vi "LoadZstackImages.vi"(0 "Experiment folder path OR Z-stack folder path":path, 11 "Error In":errorcluster) -> (1 "Number of Files":i32, 2 "All outputs":T2, 3 "AOL Z Planes":dbl[](array[numeric]), 4 "Red Image Array":T1[](array[typedef]), 6 "Green Image Array":T1[](array[typedef]), 8 "Motor Z planes":dbl[](array[numeric]), 10 "AOL Z Planes (norm)":dbl[](array[numeric]), 12 "RedMaxZ":T1, 14 "GreenMaxZ":T1, 15 "Error Out":errorcluster)   [LabVIEW 2020]
uses:
  <vilib>/vision/Image Controls.llb/IMAQ Image.ctl
  <vilib>/vision/NI_Vision_Development_Module.lvlib
panel:
  out "error IO":errorcluster
  out "Green":path[](array[path])
  out "Red":path[](array[path])
  out "GreenMaxZ":T1
  out "RedMaxZ":T1
  out "GreenImageArray":T1[](array[typedef])
  out "RedImageArray":T1[](array[typedef])
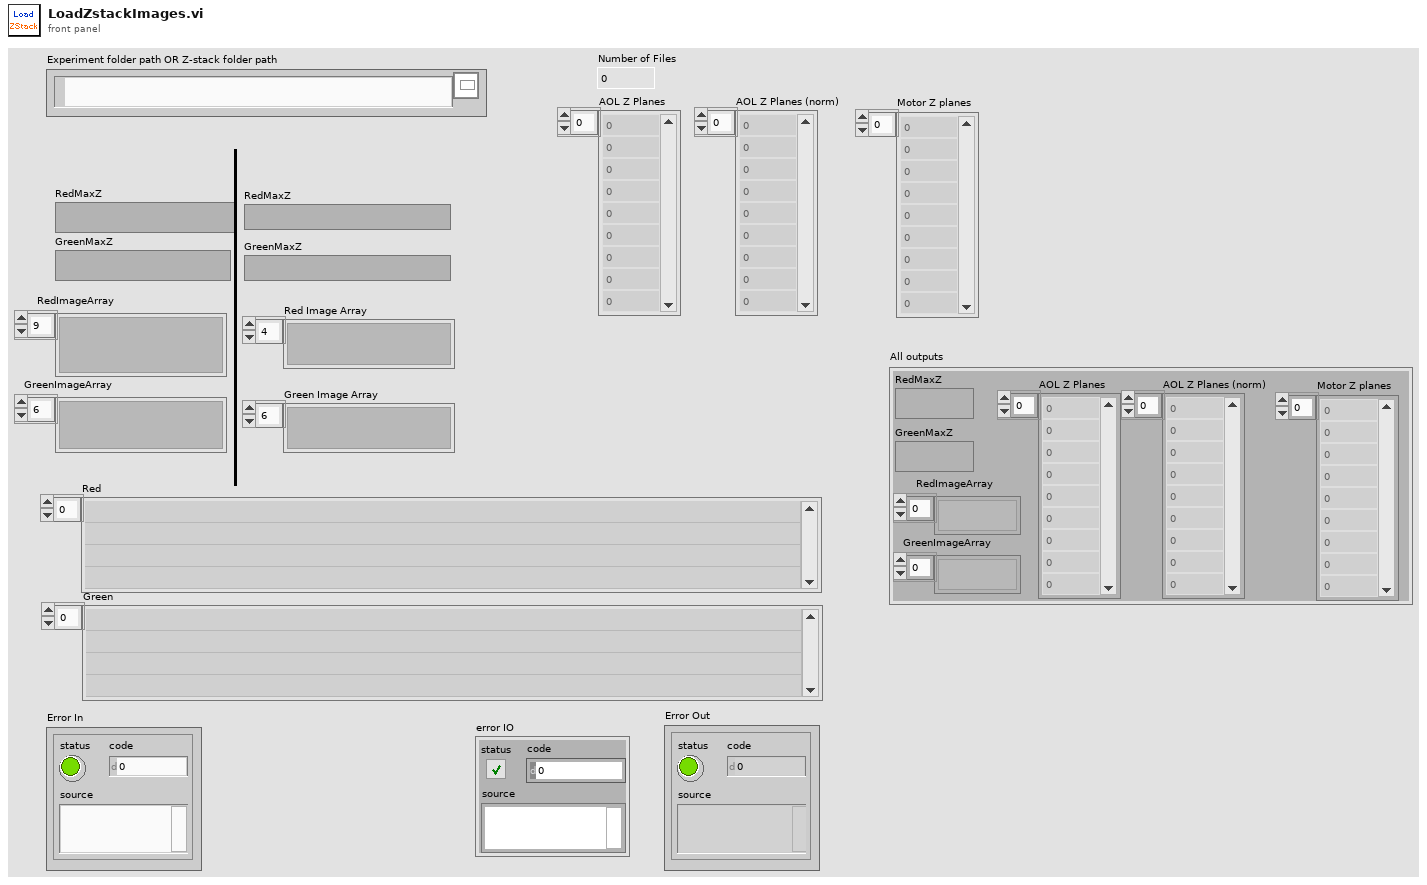
[diagram p1: front panel]
types:
  T1 = typedef "IMAQ Image.ctl" = refnum<image>
  T2 = cluster{"RedImageArray":T1[], "GreenImageArray":T1[], "RedMaxZ":T1, "GreenMaxZ":T1, "AOL Z Planes":dbl[], "AOL Z Planes (norm)":dbl[], "Motor Z planes":dbl[]}
  T3 = typedef "Fixed strings.ctl" = cluster{"ROI file name":string, "Normalised ROI file name":string, "Zplane Pockels values file name":string, "Functional data folder name":string, "Experiment Header file name":string, "Z-stack images folder name":string, "Groups setup rel. path":string, "Groups text file rel. path":string, "TDMS files folder name (F.img)":string, "TDMS files folder name (V.acq)":string, "TDMS files folder name (Pl.acq)":string, "Cycle rel times sequence file":string, "Dynamically called VIs folder name":string, "Time Series folder base name":string}
  T4 = enum32{"Average", "Min", "Max", "Clear  if < ", "Clear  if < or =", "Clear  if =", "Clear  if > or =", "Clear  if >"}
  T5 = typedef "Image Type" = u32
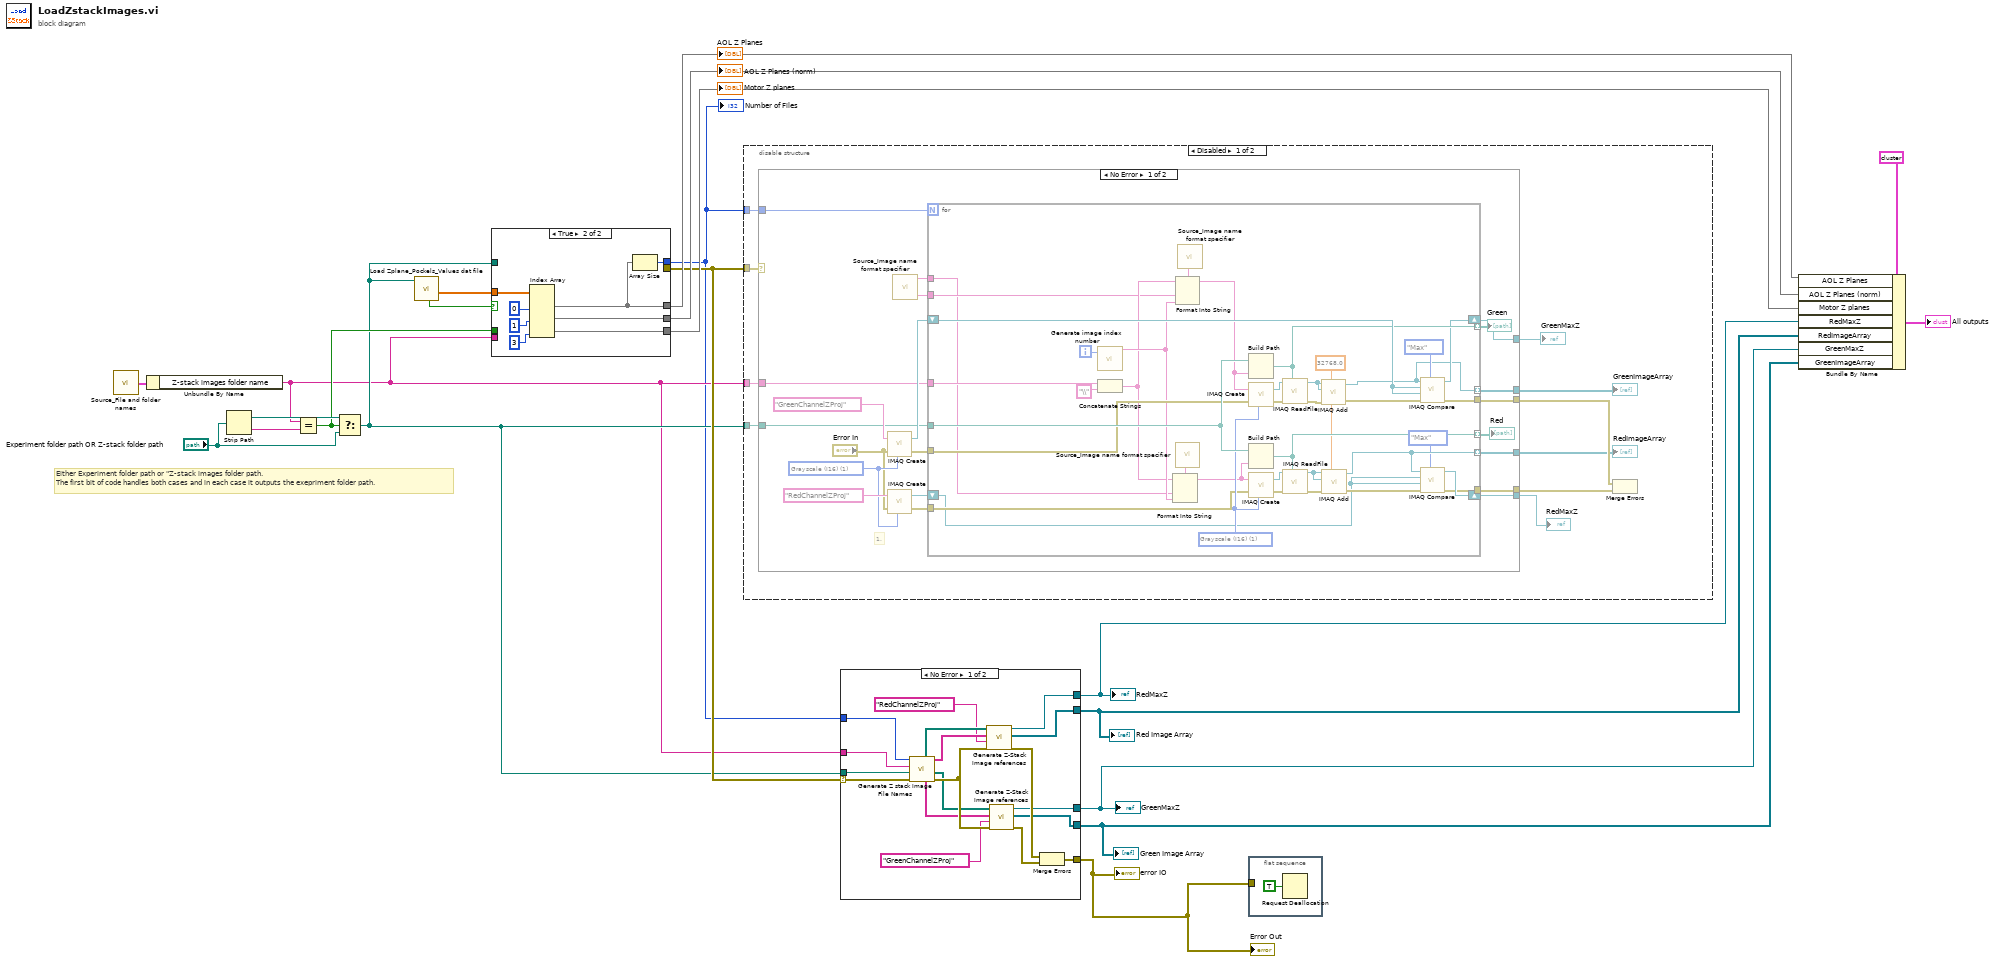
[diagram p0: block diagram]
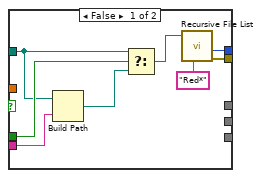
[diagram p5: hidden frame]
diagram:
  # "Either Experiment folder path or \"Z-stack images folder path.\nThe first bit of code handles both cases and in each case it outputs the exepriment folder path."
  n1 = call "Source_File and folder names.vi"() -> ("Fixed strings"=w17:T3)  [unwired: 1 in]
  n2 = Unbundle By Name(w17) -> ("Z-stack images folder name"=w7:string)
  n3 = Strip Path(path="Experiment folder path OR Z-stack folder path") -> (stripped path=w21:path, name=w19:string)
  n4 = Equal?(x=w7, y=w19) -> (x = y?=w20:bool)
  n5 = Select(t=w21, s=w20, f="Experiment folder path OR Z-stack folder path") -> (s? t:f=w8:path)
  n6 = call "Load Zplane_Pockels_Values dat file.vi"("Experiment data folder path"=w8) -> ("Zplane_Pockels_Values file data (header removed)"=w16:dbl[][], "Zplane Pockels values file exists"=w15:bool)  [unwired: 5 in, 4 out]
  n7 = case shown="True" w15 {
    tunnel: [w28 w36] -> w6
    tunnel: w8 -> [w25 _]
    tunnel: w7 -> [w27 _]
    tunnel: w20 -> [w26 _]
    tunnel: [w22 _] -> w9
    tunnel: [_ w34] -> w12
    tunnel: [_ w33] -> w11
    tunnel: w16 -> [_ w32]
    tunnel: [_ w30] -> w10
    frame False {
      n8 = Build Path(base path=w25, name or relative path=w27) -> (appended path=w24:path)
      n9 = Select(t=w25, s=w26, f=w24) -> (s? t:f=w23:path)
      n10 = call <vilib>:"Recursive File List.vi"("pattern"="Red*", "Folder Path"=w23) -> ("error out"=w22:errorcluster, "Number of Files"=w28:i32)  [unwired: 5 in, 3 out]
    }
    frame True {
      n11 = Index Array(array=w32, index (col) #1=0 ("disabled index (col)"), index (col) #2=1 ("disabled index (row)"), index (col) #3=3 ("index (col)")) -> (element #1=w34:dbl[], element #2=w33:dbl[], element #3=w30:dbl[])  [unwired: 3 in]
      n12 = Array Size(array=w34) -> (size(s)=w36:i32)
    }
  }
  "AOL Z Planes" <- w12
  "AOL Z Planes (norm)" <- w11
  "Motor Z planes" <- w10
  "Number of Files" <- w6
  n13 = disable-structure shown="Disabled" {
    disable-tunnel: w9 -> [w48 _]
    disable-tunnel: w8 -> [w47 _]
    disable-tunnel: w7 -> [w46 _]
    disable-tunnel: w6 -> [w45 _]
    frame Disabled {
      n14 = case shown="No Error" w48 {
        selector: w48 -> [_ w108]
        tunnel: [w69 _] -> w40
        tunnel: [w68 _] -> w38
        tunnel: [w59 _] -> w41
        tunnel: [w58 _] -> w44
        tunnel: [w57 w108] -> w43
        tunnel: [w56 _] -> w39
        tunnel: w45 -> [w55 _]
        tunnel: w46 -> [w54 _]
        tunnel: w47 -> [w53 _]
        frame No Error {
          w61 = T5 1 items=["Grayscale (U8)", "Grayscale (I16)", "Grayscale (SGL)", "Complex (CSG)", "RGB (U32)", "HSL (U32)", "RGB (U64)"] ("Image Type")
          # "1."
          n15 = call "IMAQ Create"("Image Name"="GreenChannelZProj" ("string"), "Image Type"=w61, "error in (no error)"="Error In") -> ("New Image"=w64:T1, "error out"=w65:errorcluster)  [unwired: 2 in]
          n16 = call "IMAQ Create"("Image Name"="RedChannelZProj" ("string"), "Image Type"=w61, "error in (no error)"="Error In") -> ("New Image"=w66:T1, "error out"=w67:errorcluster)  [unwired: 2 in]
          n17 = call "Source_Image name format specifier.vi"() -> ("Red channel name"=w50:string, "Green channel name"=w49:string)  [unwired: 5 in, 1 out]
          n18 = for {
            N: w55 -> [_]
            tunnel: [w87] -> w59 mode=indexing
            tunnel: [w70] -> w69 mode=indexing
            tunnel: w53 -> [w103]
            shift-right: [w71] -> w68
            shift-left: w64 -> [w98]
            tunnel: [w102] -> w57
            tunnel: w65 -> [w92]
            shift-right: [w101] -> w56
            shift-left: w66 -> [w83]
            tunnel: w67 -> [w91]
            tunnel: [w100] -> w58
            tunnel: w54 -> [w85]
            tunnel: [w78] -> w52 mode=indexing
            tunnel: [w75] -> w51 mode=indexing
            tunnel: w49 -> [w74]
            tunnel: w50 -> [w73]
            i -> [w96]
            w72 = 32768.0 ("Constant")
            w97 = T5 1 items=["Grayscale (U8)", "Grayscale (I16)", "Grayscale (SGL)", "Complex (CSG)", "RGB (U32)", "HSL (U32)", "RGB (U64)"] ("Image Type")
            n19 = call "Generate image index number.vi"("FOR loop iteration or existing number of files"=w96) -> ("Number in string representation (padded with zeroes)"=w81:string)  [unwired: 10 in]
            n20 = Concatenate Strings(w85, "\\" ("string")) -> (w79:string)
            n21 = call "Source_Image name format specifier.vi"() -> ("Z-Stack Image name format specifier"=w76:string)  [unwired: 5 in, 2 out]
            n22 = Format Into String(format string=w76, initial string=w79, w73, w81) -> (resulting string=w80:string)  [unwired: 1 in, 1 out]
            n23 = call "Source_Image name format specifier.vi"() -> ("Z-Stack Image name format specifier"=w77:string)  [unwired: 5 in, 2 out]
            n24 = Format Into String(format string=w77, initial string=w79, w74, w81) -> (resulting string=w82:string)  [unwired: 1 in, 1 out]
            n25 = Build Path(base path=w103, name or relative path=w82) -> (appended path=w75:path)
            n26 = call "IMAQ Create"("Image Name"=w82, "Image Type"=w97, "error in (no error)"=w92) -> ("New Image"=w105:T1, "error out"=w104:errorcluster)  [unwired: 2 in]
            n27 = Build Path(base path=w103, name or relative path=w80) -> (appended path=w78:path)
            n28 = call "IMAQ Create"("Image Name"=w80, "Image Type"=w97, "error in (no error)"=w91) -> ("New Image"=w106:T1, "error out"=w107:errorcluster)  [unwired: 2 in]
            n29 = call "IMAQ ReadFile"("File Path"=w75, "error in (no error)"=w104, "Image"=w105) -> ("error out"=w93:errorcluster, "Image Out"=w95:T1)  [unwired: 4 in, 3 out]
            n30 = call "IMAQ ReadFile"("File Path"=w78, "error in (no error)"=w107, "Image"=w106) -> ("error out"=w90:errorcluster, "Image Out"=w94:T1)  [unwired: 4 in, 3 out]
            n31 = call "IMAQ Add"("Image Src A"=w95, "Constant"=w72, "Image Dst"=w95, "error in (no error)"=w93) -> ("Image Dst Out"=w70:T1, "error out"=w88:errorcluster)  [unwired: 3 in]
            n32 = call "IMAQ Add"("Image Src A"=w94, "Constant"=w72, "Image Dst"=w94, "error in (no error)"=w90) -> ("Image Dst Out"=w87:T1, "error out"=w89:errorcluster)  [unwired: 3 in]
            n33 = call "IMAQ Compare"("Operator"=T4."Max", "error in (no error)"=w88, "Image Src B"=w98, "Image Dst"=w98, "Image Src A"=w70) -> ("error out"=w102:errorcluster, "Image Dst Out"=w71:T1)  [unwired: 5 in]
            n34 = call "IMAQ Compare"("Operator"=T4."Max", "error in (no error)"=w89, "Image Src B"=w83, "Image Dst"=w83, "Image Src A"=w87) -> ("error out"=w100:errorcluster, "Image Dst Out"=w101:T1)  [unwired: 5 in]
          }
          "Red" <- w52
          "Green" <- w51
        }
        frame Error {
        }
      }
      "RedImageArray" <- w41
      "GreenImageArray" <- w40
      "RedMaxZ" <- w39
      "GreenMaxZ" <- w38
      n35 = Merge Errors(w43, w44) -> (w42:errorcluster)
    }
    frame Enabled {
    }
  }
  n36 = case shown="No Error" w9 {
    selector: w9 -> [w123 w127]
    tunnel: w8 -> [w126 _]
    tunnel: w7 -> [w125 _]
    tunnel: w6 -> [w124 _]
    tunnel: [w114 _] -> w5
    tunnel: [w113 _] -> w4
    tunnel: [w112 _] -> w3
    tunnel: [w111 _] -> w2
    tunnel: [w110 w127] -> w1
    frame No Error {
      n37 = call "Generate Z stack Image File Names.vi"("error in (no error)"=w123, "Z Stack Image Folder Path"=w126, "Z Stage Image Folder Name"=w125, "Z Stack Size"=w124) -> ("error out"=w122:errorcluster, "Green Channel File Paths"=w119:path[], "Red Channel Image Names"=w121:string[], "Green Channel Image Names"=w109:string[], "Red Channel File Paths"=w120:path[])  [unwired: 3 in]
      n38 = call "Generate Z-Stack Image references.vi"("error in (no error)"=w122, "IMAQ reference name"="RedChannelZProj" ("string"), "Channel File Names"=w121, "Channel File Paths"=w120) -> ("error out"=w115:errorcluster, "Image Array refs"=w113:T1[], "MaxZ"=w114:T1)  [unwired: 5 in]
      n39 = call "Generate Z-Stack Image references.vi"("error in (no error)"=w122, "IMAQ reference name"="GreenChannelZProj" ("string"), "Channel File Names"=w109, "Channel File Paths"=w119) -> ("error out"=w116:errorcluster, "Image Array refs"=w111:T1[], "MaxZ"=w112:T1)  [unwired: 5 in]
      n40 = Merge Errors(w115, w116) -> (w110:errorcluster)
    }
    frame Error {
    }
  }
  "Error Out" <- w1
  "Red Image Array" <- w4
  "RedMaxZ" <- w5
  "Green Image Array" <- w2
  "GreenMaxZ" <- w3
  "error IO" <- w1
  n41 = flat-sequence {
    tunnel: w1 -> [_]
    frame #0 {
      n42 = Request Deallocation(TRUE ("flag")) -> ()
    }
  }
  n43 = Bundle By Name(cluster=T2 {"RedImageArray"=[], "GreenImageArray"=[], "RedMaxZ"=refnum, "GreenMaxZ"=refnum, "AOL Z Planes"=[], "AOL Z Planes (norm)"=[], "Motor Z planes"=[]} ("All outputs"), "AOL Z Planes"=w12, "AOL Z Planes (norm)"=w11, "Motor Z planes"=w10, "RedMaxZ"=w5, "RedImageArray"=w4, "GreenMaxZ"=w3, "GreenImageArray"=w2) -> (→"All outputs":T2)
